vi "LinearFit.vi"(5 "End":dbl, 7 "Start":dbl, 10 "10/20":bool, 11 "Data Cluster":T1) -> (0 "X":dbl[](array[numeric]), 1 "intercept":dbl, 2 "Best Linear Fit":dbl[](array[numeric]), 3 "slope":dbl, 4 "Y":dbl[](array[numeric]))   [LabVIEW 2020]
uses:
  controls/UI Data.ctl
  <vilib>/Analysis/NI_AALPro.lvlib
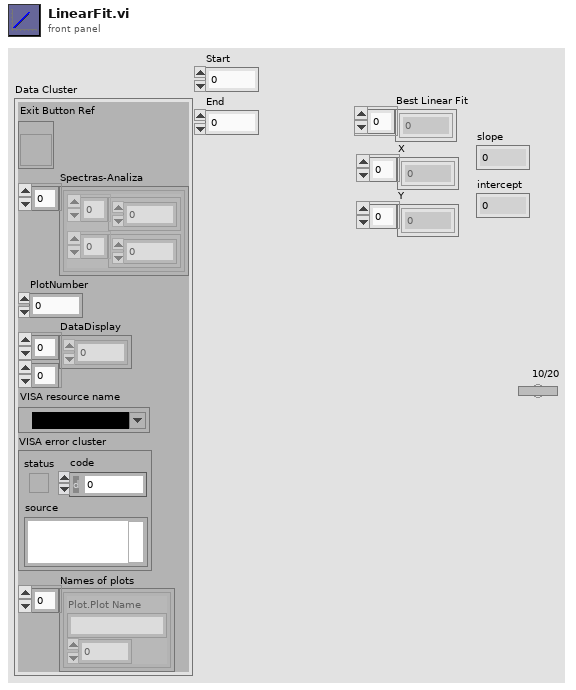
[diagram p1: front panel]
types:
  T1 = typedef "UI Data.ctl" = cluster{"Exit Button Ref":refnum<vi>, "Spectras-Analiza":cluster{dbl[], dbl[]}[], "PlotNumber":dbl, "DataDisplay":dbl[][], "VISA resource name":refnum<visa-resource-name>, "VISA error cluster":errorcluster, "Names of plots":cluster{"Plot.Plot Name":string, i32}[]}
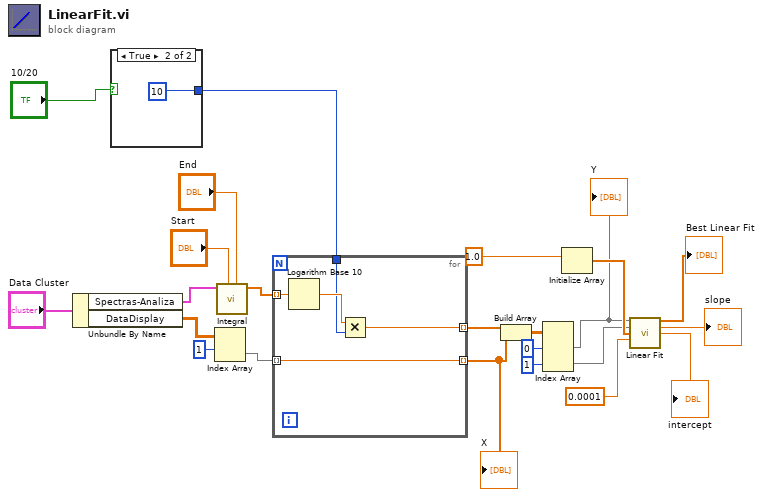
[diagram p0: block diagram]
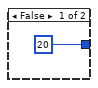
[diagram p2: hidden frame]
diagram:
  n1 = Unbundle By Name("Data Cluster") -> ("Spectras-Analiza"=w20:cluster{dbl[], dbl[]}[], "DataDisplay"=w22:dbl[][])
  n2 = case shown="True" "10/20" {
    tunnel: [20 10] -> w1
    frame False {
    }
    frame True {
    }
  }
  n3 = Index Array(array=w22, index (row)=1) -> (element=w14:dbl[])  [unwired: 1 in]
  n4 = call "Integral.vi"("End"="End", "Start"="Start", "Spectras-Analiza"=w20) -> ("Integral"=w19:dbl[])  [unwired: 8 in]
  n5 = for {
    tunnel: w19 -> [w29] mode=indexing
    tunnel: [w28] -> w13 mode=indexing
    tunnel: w14 -> [w27] mode=indexing
    tunnel: [w27] -> w3 mode=indexing
    tunnel: w1 -> [w26]
    n6 = Logarithm Base 10(1:w29) -> (0:w30:dbl)
    n7 = Multiply(x=w30, y=w26) -> (x*y=w28:dbl)
  }
  "X" <- w3
  n8 = Build Array(w13, w3) -> (w12:dbl[][])
  n9 = Index Array(array=w12, index (row) #1=0 ("index (row)"), index (row) #2=1 ("index (row)")) -> (element #1=w9:dbl[], element #2=w8:dbl[])  [unwired: 2 in]
  "Y" <- w9
  n10 = Initialize Array(1.0 ("element")) -> (w15:dbl[])  [unwired: 1 in]
  n11 = call <vilib>:"Linear Fit.vi"("Y"=w9, "X"=w8, "Weight"=w15, "tolerance"=0.0001) -> ("Best Linear Fit"=→"Best Linear Fit":dbl[], "slope"=→"slope":dbl, "intercept"=→"intercept":dbl)  [unwired: 7 in, 2 out]
